vi "Untitled 1.vi"() -> ()   [LabVIEW 2020]
uses:
  <vilib>/userdefined/High Color/IMAQdx.ctl
  <vilib>/vision/driver/NI_Vision_Acquisition_Software.lvlib
panel:
  out "Status":bool
  out "Detected sign":string
  out "Python Error Out":errorcluster
  in  "Off/On":bool caption="Start/Stop Vision"
  out "error out 4":errorcluster
  out "Live view":T1(plugin-control)
  out "Camera Status":errorcluster
  in  "Exit program":bool
  out "IMAQ Err":errorcluster
  in  "Camera Device":T2="cam0"
  # "Vision control panel"
  # "Camera configuration"
  # "Error section"
  # "Tymczasowe"
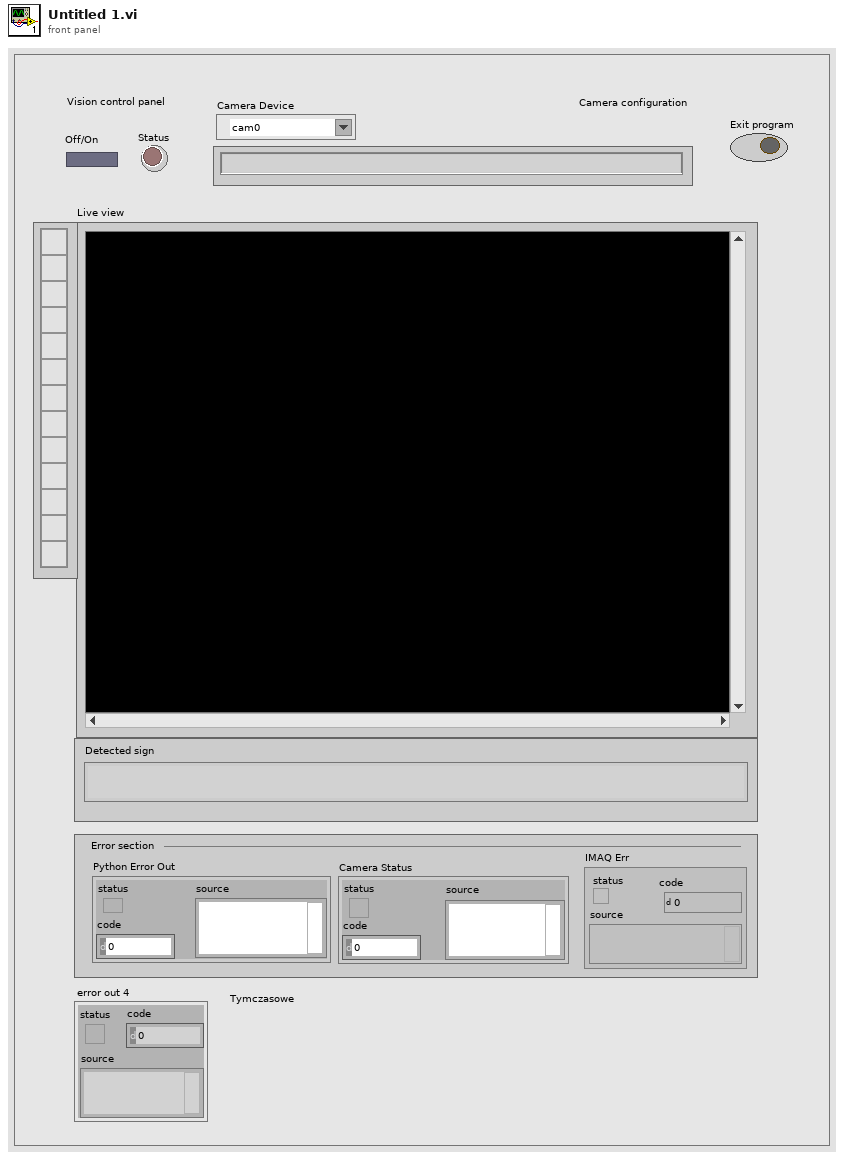
[diagram p1: front panel]
types:
  T1 = typedef "IMAQ Image.ctl" = refnum<image>
  T2 = typedef "IMAQdx.ctl" = refnum<k21>
  T3 = typedef "Image Type" = u32
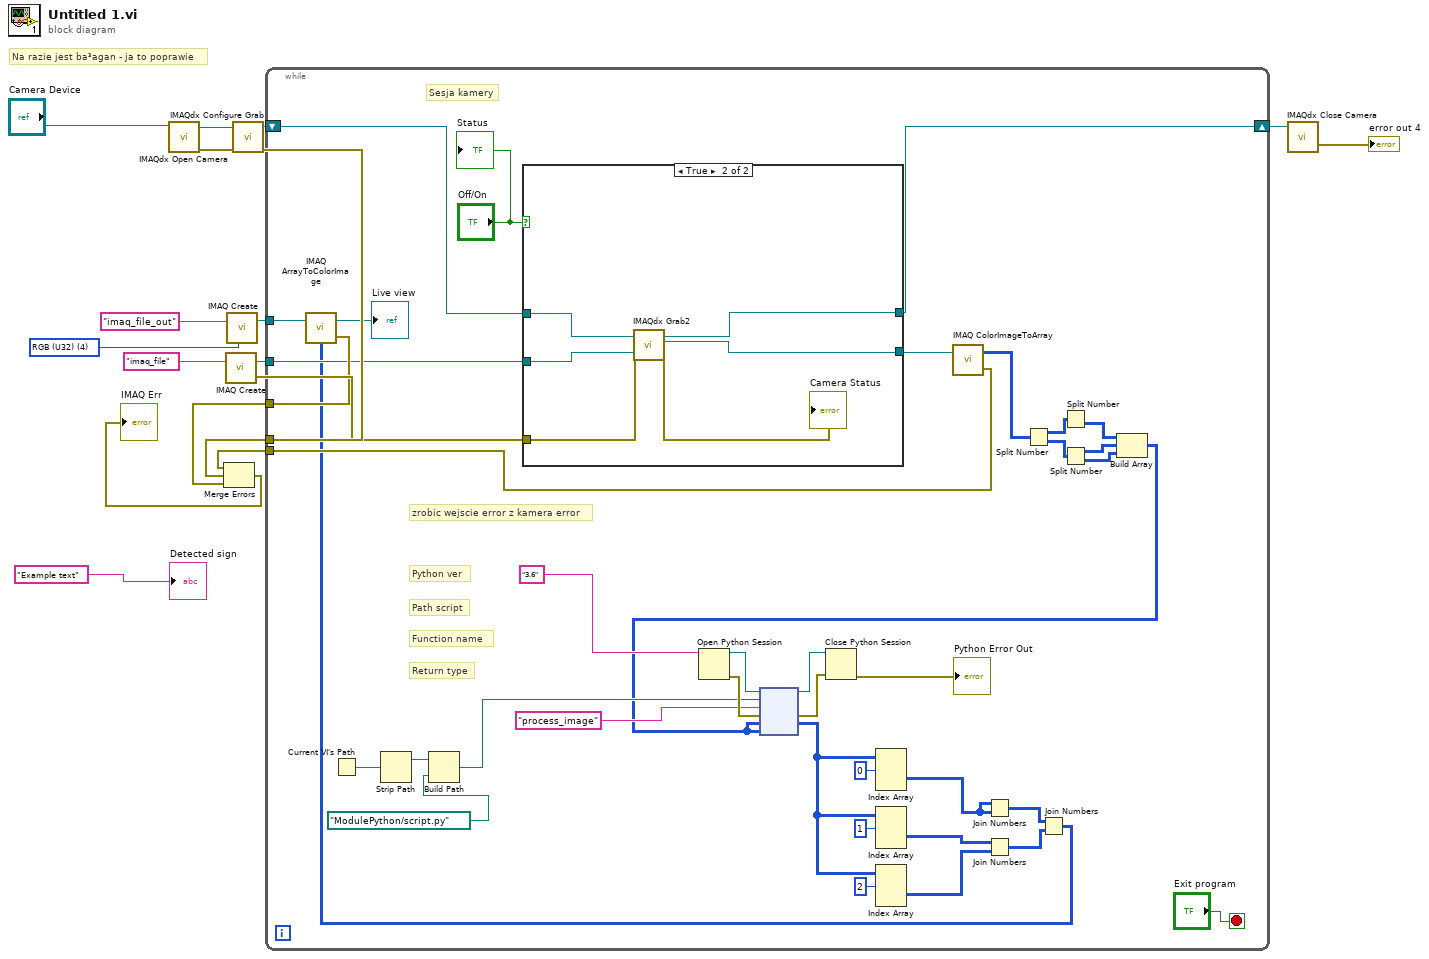
[diagram p0: block diagram]
diagram:
  w1 = T3 4 items=["Grayscale (U8)", "Grayscale (I16)", "Grayscale (SGL)", "Complex (CSG)", "RGB (U32)", "HSL (U32)", "RGB (U64)", "Grayscale (U16)"] ("Image Type")
  # "Na razie jest ba³agan - ja to poprawie"
  n1 = call <vilib>:"IMAQdx Open Camera.vi"("Session In"="Camera Device") -> ("error out"=w12:errorcluster, "Session Out"=w11:T2)  [unwired: 9 in]
  n2 = call "IMAQ Create"("Image Name"="imaq_file") -> ("New Image"=w16:T1, "error out"=w6:errorcluster)  [unwired: 4 in]
  n3 = call "IMAQ Create"("Image Name"="imaq_file_out", "Image Type"=w1) -> ("New Image"=w2:T1)  [unwired: 3 in, 1 out]
  n4 = call <vilib>:"IMAQdx Configure Grab.vi"("error in"=w12, "Session In"=w11) -> ("error out"=w17:errorcluster, "Session Out"=w15:T2)  [unwired: 8 in]
  n5 = while {
    tunnel: w16 -> [w36]
    shift-right: [w53] -> w14
    shift-left: w15 -> [w54]
    tunnel: w17 -> [w55]
    tunnel: [w44] -> w7
    tunnel: [w39] -> w4
    tunnel: w2 -> [w35]
    stop <- "Exit program" stop-if-true
    # "Function name"
    # "zrobic wejscie error z kamera error"
    # "Python ver"
    # "Path script"
    # "Return type"
    # "Sesja kamery"
    n6 = Current VI's Path() -> (path=w43:path)
    n7 = Strip Path(path=w43) -> (stripped path=w42:path)  [unwired: 1 out]
    n8 = Build Path(base path=w42, name or relative path=path "ModulePython/script.py" ("module path")) -> (appended path=w40:path)
    n9 = case shown="True" "Off/On" {
      tunnel: w55 -> [_ w63]
      tunnel: w54 -> [w58 w62]
      tunnel: w36 -> [w57 w61]
      tunnel: [w58 w60] -> w53
      tunnel: [w57 w59] -> w38
      frame False {
      }
      frame True {
        n10 = call <vilib>:"IMAQdx Grab2.vi"("error in"=w63, "Image In"=w61, "Session In"=w62) -> ("error out"=→"Camera Status":errorcluster, "Image Out"=w59:T1, "Session Out"=w60:T2)  [unwired: 5 in, 1 out]
      }
    }
    n11 = Open Python Session(python version="3.6") -> (session out=w51:refnum<k35>, error out=w48:errorcluster)  [unwired: 2 in]
    n12 = call "IMAQ ColorImageToArray"("Image"=w38) -> ("Image Pixels (U32)"=w32:u32[][], "error out"=w44:errorcluster)  [unwired: 3 in, 1 out]
    n13 = Split Number(x=w32) -> (hi(x)=w34:u16[][], lo(x)=w33:u16[][])
    n14 = Split Number(x=w34) -> (lo(x)=w29:u8[][])  [unwired: 1 out]
    n15 = Split Number(x=w33) -> (hi(x)=w30:u8[][], lo(x)=w31:u8[][])
    n16 = Build Array(w29, w30, w31) -> (w28:u8[][][])
    n17 = node(w51, w40, "process_image" ("function name"), w48, w28, w28) -> (w50:refnum<k35>, w47:errorcluster, w27:u8[][][])  [unwired: 1 in, 2 out]
    n18 = Close Python Session(session in=w50, error in=w47) -> (11:→"Python Error Out":errorcluster)
    n19 = Index Array(array=w27, index (dim 0)=0 ("index (page)")) -> (element=w18:u8[][])  [unwired: 2 in]
    n20 = Index Array(array=w27, index (dim 0)=1 ("index (page)")) -> (element=w21:u8[][])  [unwired: 2 in]
    n21 = Index Array(array=w27, index (dim 0)=2 ("index (page)")) -> (element=w20:u8[][])  [unwired: 2 in]
    n22 = Join Numbers(hi=w18, lo=w18) -> ((hi.lo)=w23:u16[][])
    n23 = Join Numbers(hi=w21, lo=w20) -> ((hi.lo)=w22:u16[][])
    n24 = Join Numbers(hi=w23, lo=w22) -> ((hi.lo)=w19:u32[][])
    n25 = call "IMAQ ArrayToColorImage"("Image Pixels (U32)"=w19, "Image"=w35) -> ("Image Out"=→"Live view":T1, "error out"=w39:errorcluster)  [unwired: 3 in]
    "Status" <- "Off/On"
  }
  n26 = Merge Errors(w7, w6, w4) -> (→"IMAQ Err":errorcluster)
  n27 = call <vilib>:"IMAQdx Close Camera.vi"("Session In"=w14) -> ("error out"=→"error out 4":errorcluster)  [unwired: 10 in]
  "Detected sign" <- "Example text"
